vi "getFPGA.vi"(11 "ModbusIRQ in":refnum<class "ModbusIRQ.lvclass">) -> (2 "FPGA":refnum<class "FPGA.lvclass">, 3 "ModbusIRQ out":refnum<class "ModbusIRQ.lvclass">)   [LabVIEW 2016, in "ModbusIRQ.lvclass"]
uses:
  ModbusIRQ.lvclass
  FPGA/FPGA.lvclass
  ModbusIRQ.lvclass/ModbusIRQ.ctl
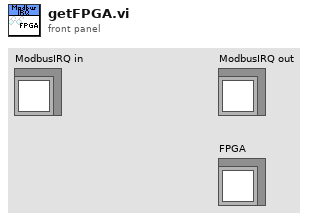
[diagram p1: front panel]
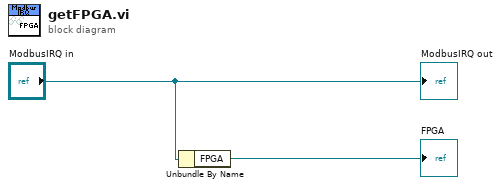
[diagram p0: block diagram]
diagram:
  n1 = Unbundle By Name("ModbusIRQ in") -> ("FPGA"=→"FPGA":refnum<class "FPGA.lvclass">)
  "ModbusIRQ out" <- "ModbusIRQ in"
